vi "play-batch-raster-scan.vi"() -> ()   [LabVIEW 2017]
uses:
  raster-scan-params.ctl
  controls/PI-params.ctl
  controls/boolean_info.ctl
  controls/raster_input_meta_data.ctl
  <vilib>/userdefined/High Color/nirio_resource_hc.ctl
  controls/rasterMetaData.ctl
  <vilib>/FPGAPlugInAG/cRIO-9082/niLvFpga_Open_cRIO-9082.vi
  <vilib>/rvi/interface/common/dynamic/niFpgaDynamicAddResources.vi
  <vilib>/FPGAPlugInAG/Dynamic/niLvFpga_Reset_Dynamic.vi
  <vilib>/rvi/interface/common/niFpgaWaitOnOcc.vi
  <vilib>/Utility/error.llb/Error Cluster From Error Code.vi
  <vilib>/rvi/errors/niLvFpgaAdjustHostInterfaceError.vi
  <vilib>/FPGAPlugInAG/Dynamic/niLvFpga_Run_Dynamic.vi
  <vilib>/Utility/file.llb/Read Delimited Spreadsheet (DBL).vi
  <vilib>/FPGAPlugInAG/Dynamic/niLvFpga_Close_Dynamic.vi
  <userlib>/_matio/level5/Public/Write/Append Data Element.llb/Append Data Element (Anything).vi
  <vilib>/rvi/interface/nirviOpenFPGA/nirviOpenFPGA.xnode
  FPGA Bitfiles/afmimagingcontro_FPGATargetSPARTA_raster-scanning_DXF4O8EAjZ4.lvbitx
  <vilib>/rvi/interface/nirviMethod/nirviMethod.xnode
  <vilib>/rvi/interface/nirviReadWriteControl/nirviReadWriteControl.xnode
  <vilib>/rvi/interface/nirviCloseFPGA/nirviCloseFPGA.xnode
  <vilib>/FPGAPlugInAG/Dynamic/niLvFpga_ConfigureFifo_Dynamic.vi
  <vilib>/rvi/errors/niLvFpgaMergeErrorWithErrorCode.vi
  <vilib>/rvi/interface/Simulation/niFpgaSimulationCallBeginRW.vi
  <vilib>/FPGAPlugInAG/Dynamic/niLvFpga_ReadFifo_Dynamic.vi
  fpga_interface_lib/fpga_interface.lvlib
  NiFpgaLv.dll
  <userlib>/_matio/level5.lvlib
  <vilib>/FPGAPlugInAG/Dynamic/niLvFpga_WriteFifo_Dynamic.vi
panel:
  in  "Input-files":path[](array[path])
  out "Array 2":path[](array[path])
  out "control":dbl[](graph)
  out "error":dbl[](graph)
  out "InputMetaData":T1
  out "output-meta-data-path":path
  in  "Tab Control":enum32{"Page 1", "Debug"}(tab)
  in  "number-of-pixels":i32=256
  out "points_per_line":i32=250000
  out "total_num_points":i32
  in  "raise-constant (init)":sgl
  in  "raise-constant":sgl
  in  "trigger-0":bool
  in  "STOP":bool
  in  "xy-init":fxp<+/-,16,5>[](array[numeric])=[0.0, 0.0]
  in  "Ki-xy":dbl=0.01 format="%#_13g"
  out "ADC-zaxis":sgl
  out "DAC-zaxis":sgl
  in  "xy-bound":sgl=7.0
  out "current_output-data-path":path
  in  "note-blob":string
  in  "overwrite":bool
  in  "raster-scan-params":T2={"TsTicks"=1600, "Stop"=FALSE, "TOL"=0.3, "ramp-rate"=-5e-05, "z-u-max"=5.0, "PI-params"={"Ki"=0.01, "setpoint"=0.0}, "Num"=[1.0, 0.0, 0.0, 0.0, 0.0, 0.0, 0.0, 0.0, 0.0], "TF Order"=1, "Den"=[1.0, 0.0, 0.0, 0.0, 0.0, 0.0, 0.0, 0.0, 0.0]} {"ramp-rate" format="%#_5g"; "TOL" format="%#_13g"}
  in  "do-Dz":bool
  in  "do_xy_CL":bool
  out "boolean errors":T4
  in  "Z-settle-N":i16=10000
  out "Actual Depth":u32
  out "Elements Remaining":u32
  out "size(s)":i32
  out "y iter":i32
  out "nsamps 2":i32
  out "Empty Elements Remaining":u32
  out "(int) y*floor(x/y)":u64
  out "elements left 2":i32=1
  out "x >= y?":bool
  out "writing stopped":bool
  out "size(s) 2":i32
  out "case-selector-feedback":i16
  out "e(0) (threshhold init)":fxp<+/-,16,5>
  out "total-time":dbl
  out "x+1":i32
  out "que timed out?":bool
  out "Error signal (previous line) 2":dbl[](graph)
  out "Waveform Graph":dbl[](graph)
  out "base y_ref (ramp)":dbl[](graph)
  out "base x_ref(triangle wave)":dbl[](graph)
  out "Intensity Graph":dbl[][](graph)
  out "Error signal (previous line)":dbl[](graph)
  # "x-axis"
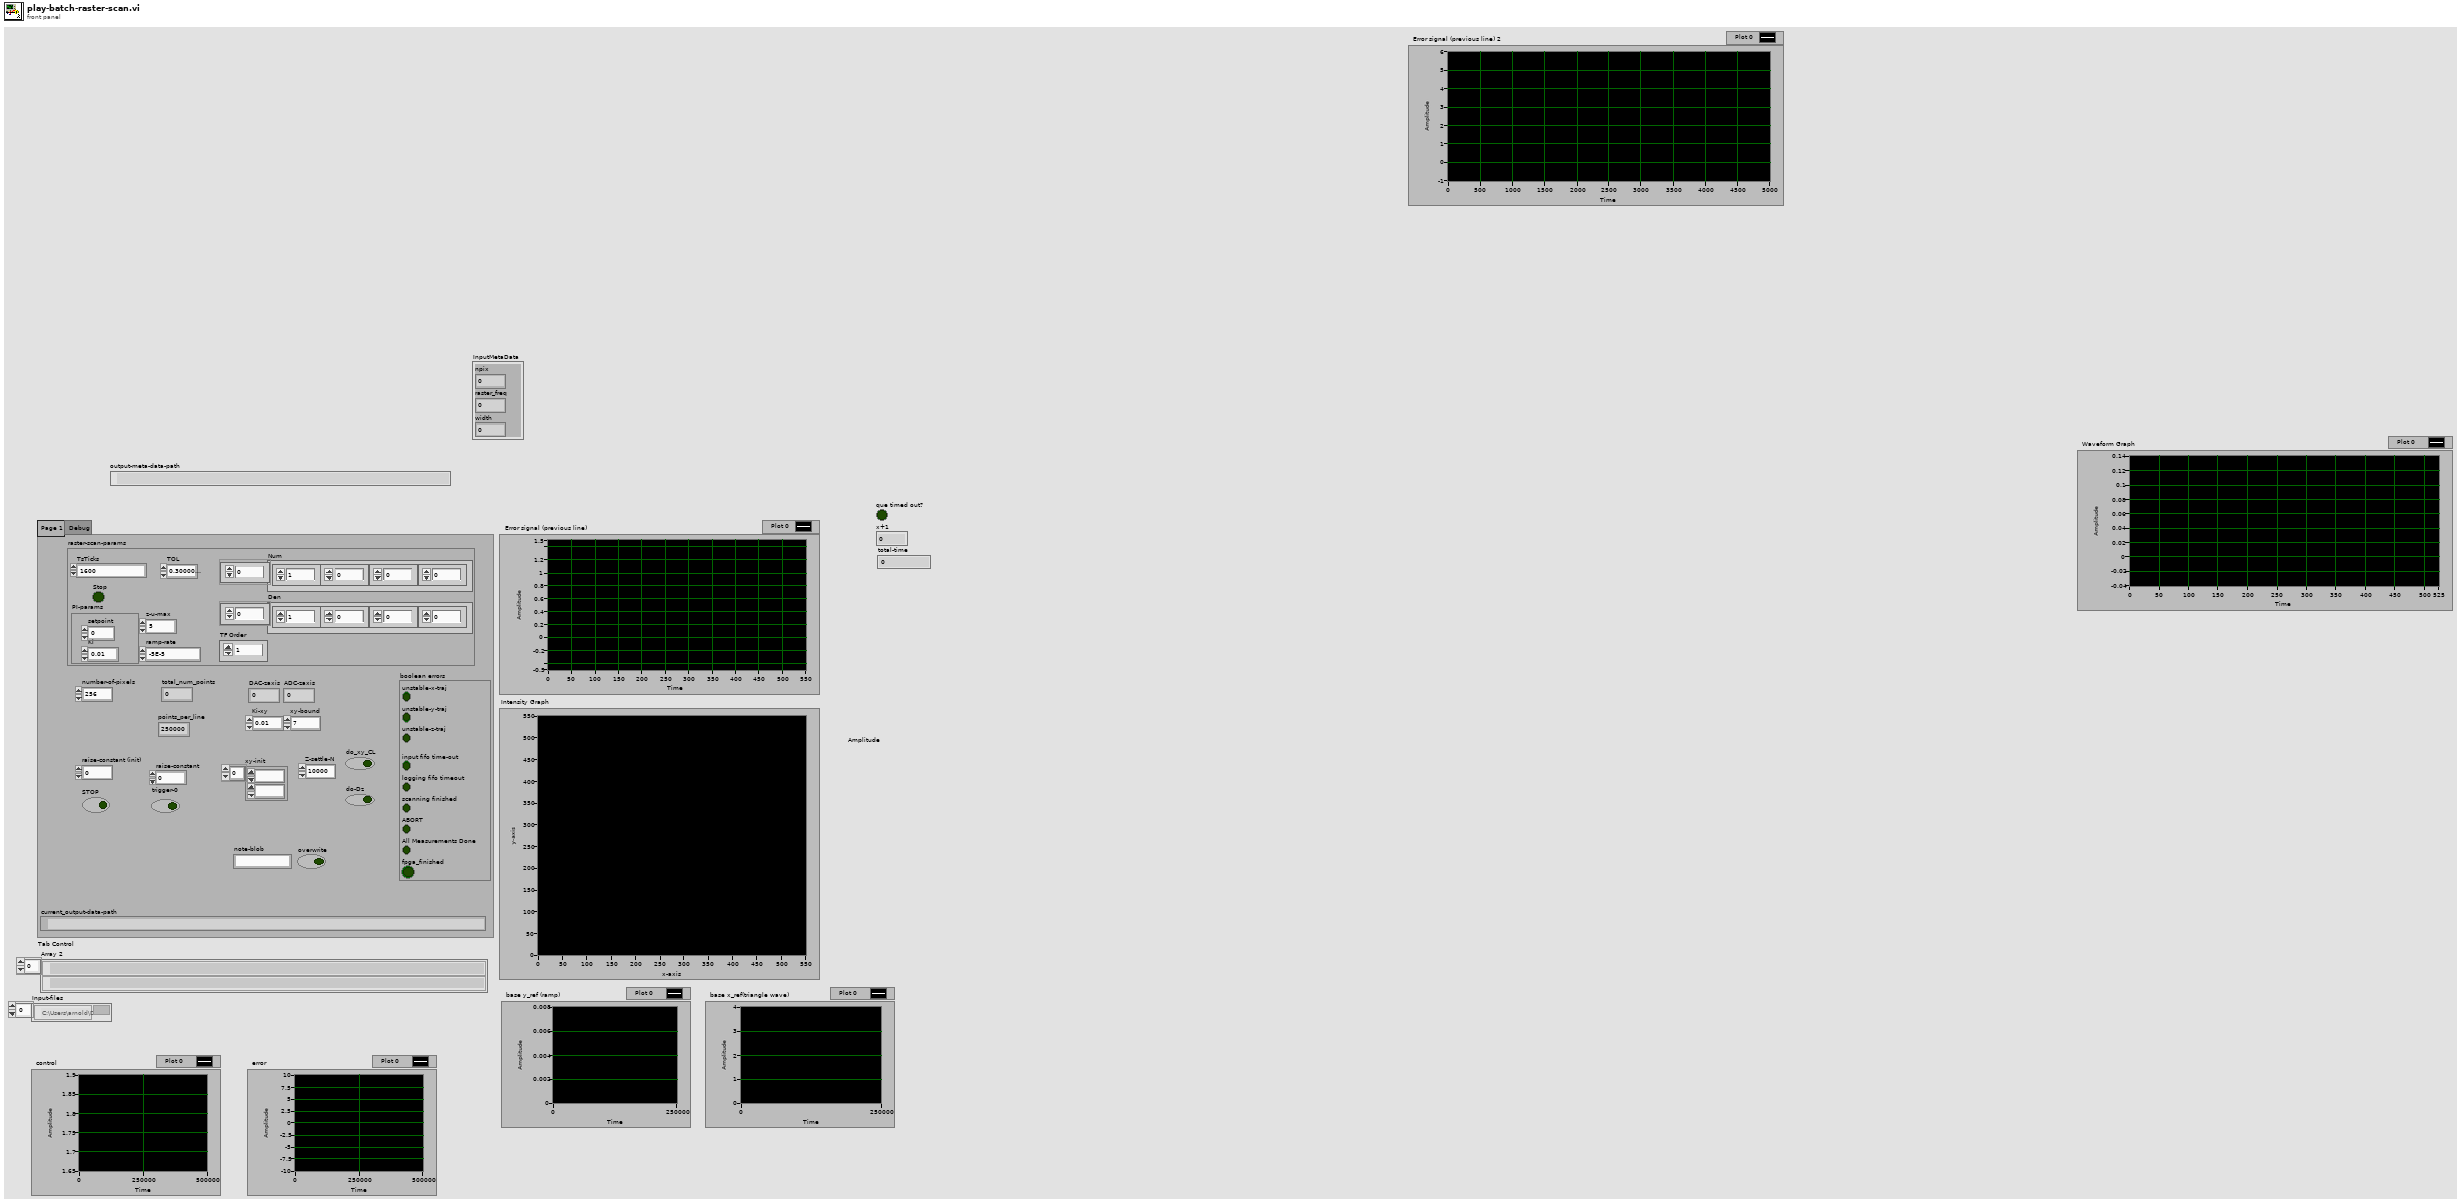
[diagram p1: front panel]
types:
  T1 = typedef "raster_input_meta_data.ctl" = cluster{"npix":dbl, "raster_freq":dbl, "width":dbl}
  T2 = typedef "raster-scan-params.ctl" = cluster{"TsTicks":u32, "Stop":bool, "TOL":sgl, "ramp-rate":sgl, "z-u-max":sgl, "PI-params":T3, "Num":sgl[], "TF Order":i32, "Den":sgl[]}
  T3 = typedef "PI-params.ctl" = cluster{"Ki":sgl, "setpoint":sgl}
  T4 = typedef "boolean_info.ctl" = cluster{"unstable-z-traj":bool, "input fifo time-out":bool, "logging fifo timeout":bool, "scanning finished":bool, "unstable-x-traj":bool, "unstable-y-traj":bool, "ABORT":bool, "All Measurements Done":bool, "fpga_finished":bool}
  T5 = typedef "nirio_resource_hc.ctl" = tag
  T6 = typedef "rasterMetaData.ctl" = cluster{"raster-scan-params":T2, "xy-bound":sgl, "DAC-zaxis":sgl, "ADC-zaxis":sgl, "Ki-xy":dbl, "total_num_points":i32, "points_per_line":i32, "number-of-lines":i32, "number-of-pixels":i32, "raster_meta_in":T1, "Ki-derate":sgl, "ze_sched_thresh":sgl}
  T7 = enum16{"open", "replace", "create", "open or create", "replace or create", "replace or create with confirmation"}
  T8 = cluster{"unstable-z-traj":bool, "input fifo time-out":bool, "logging fifo timeout":bool, "scanning finished":bool, "unstable-x-traj":bool, "unstable-y-traj":bool, "ABORT":bool, "All Measurements Done":bool, "fpga_finished":bool}
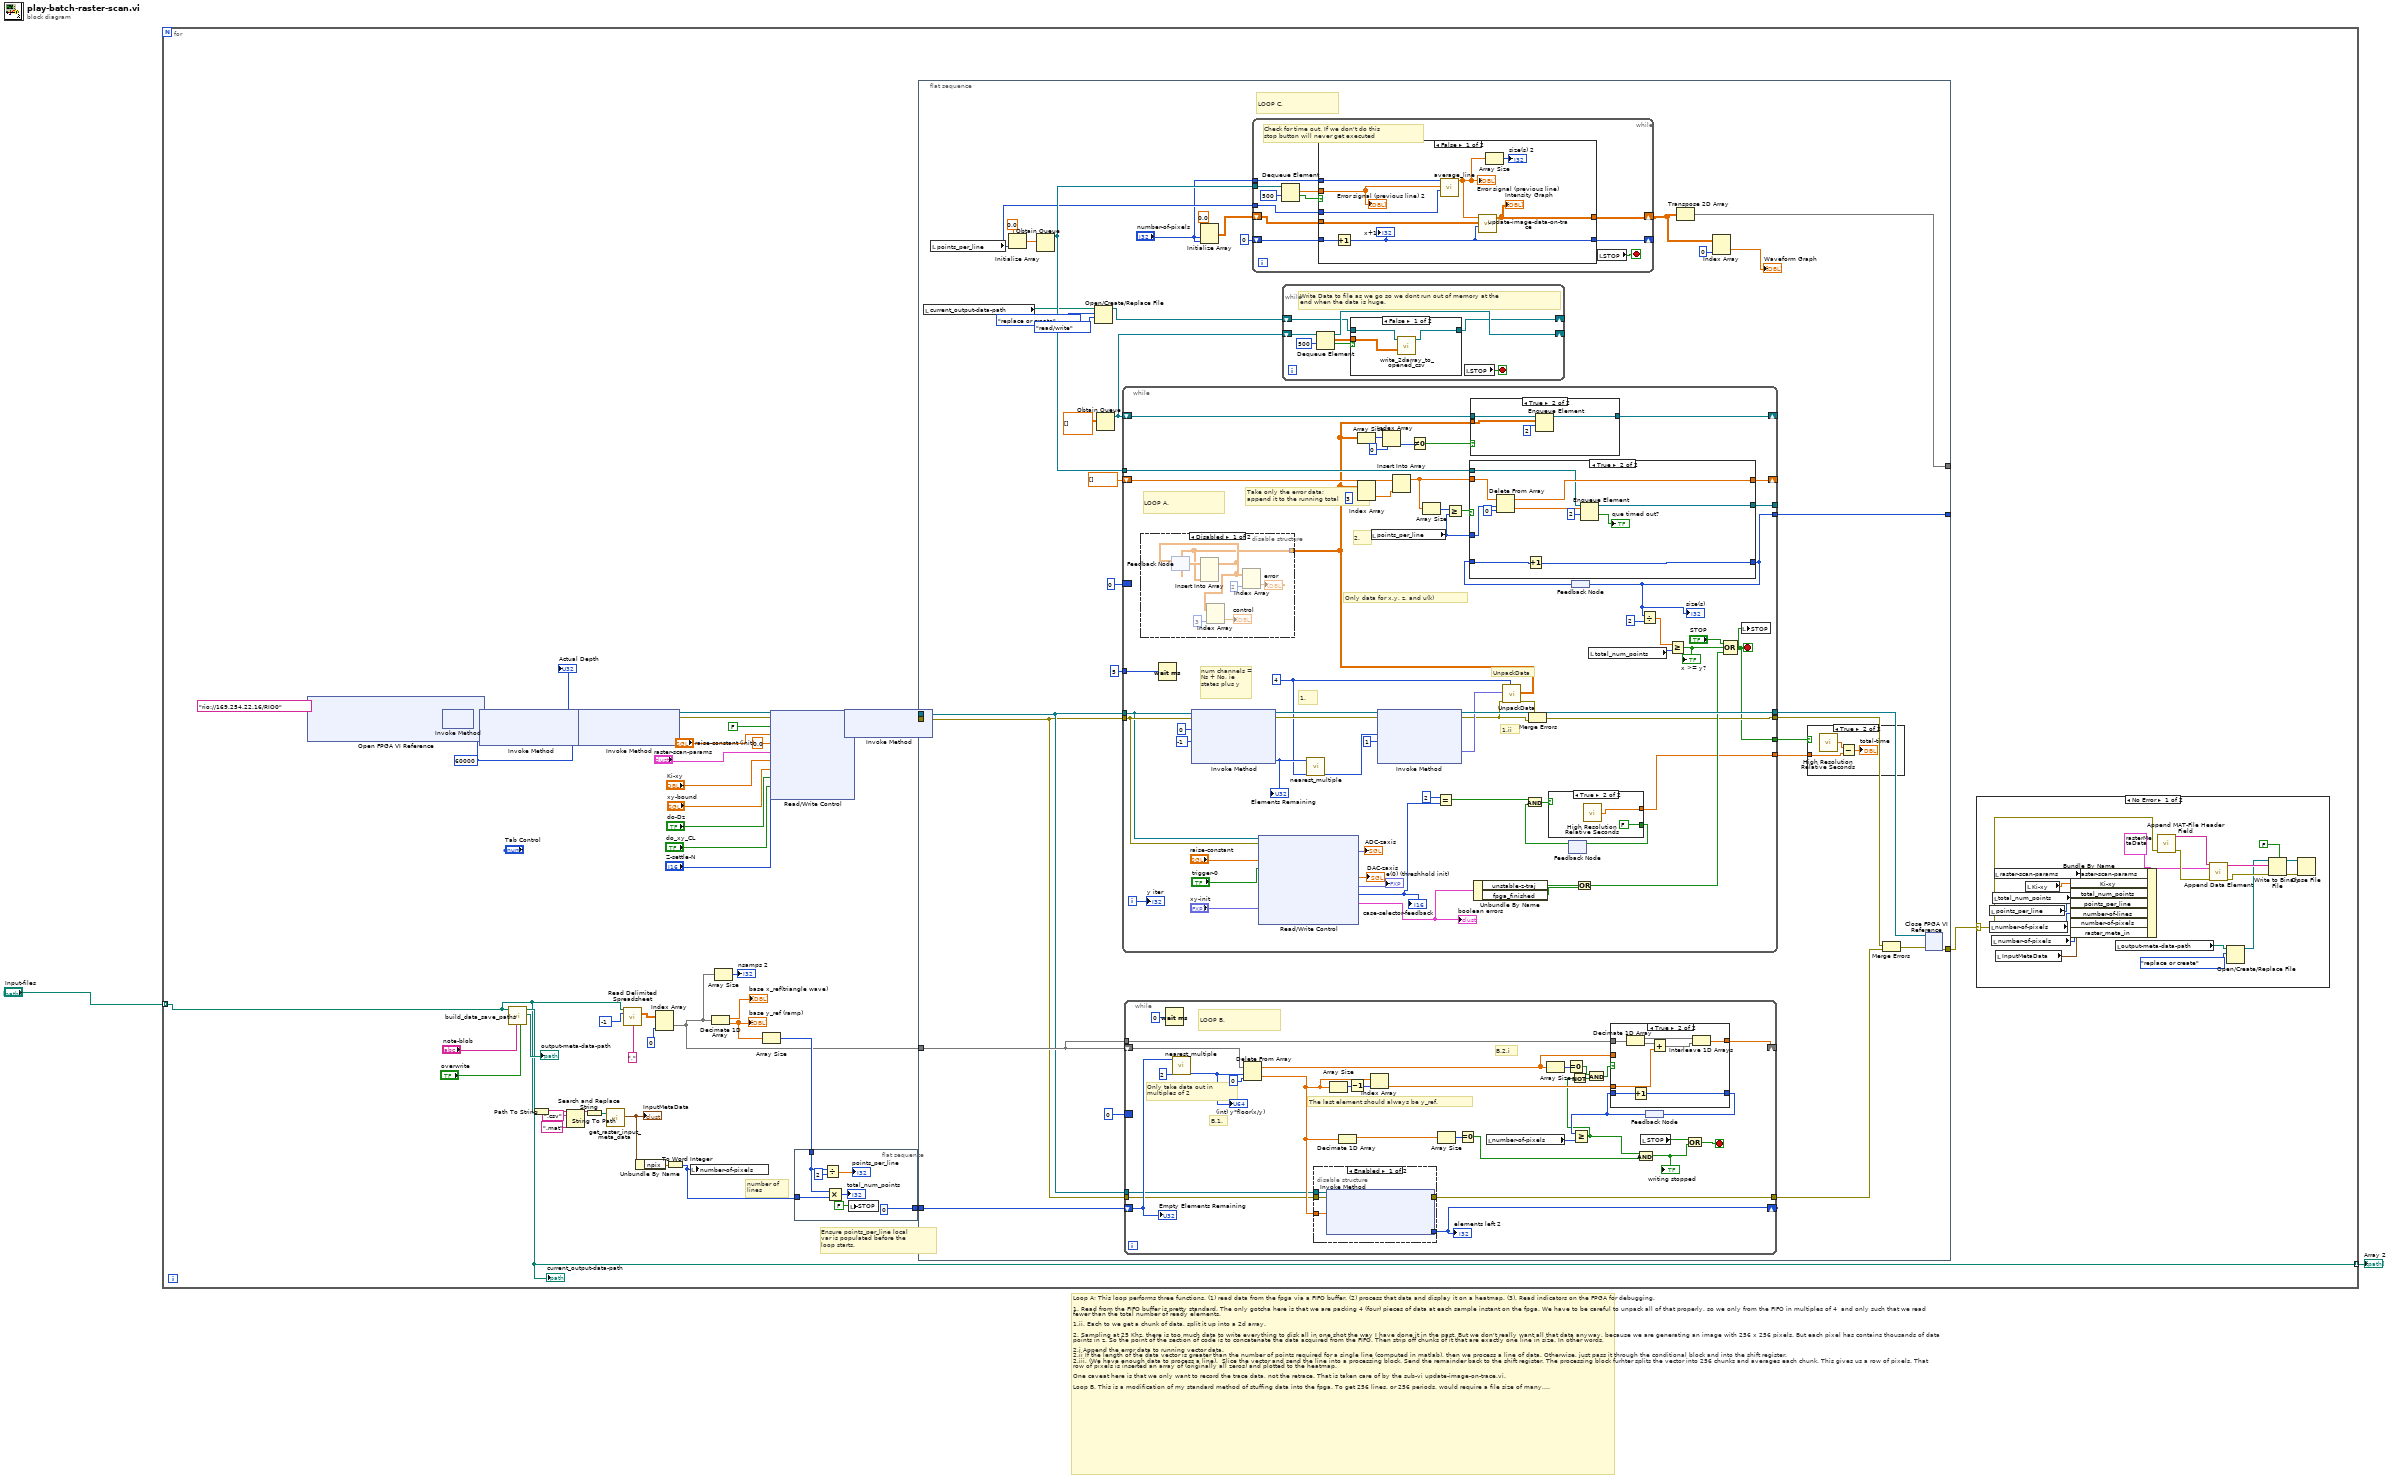
[diagram p0: block diagram]
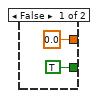
[diagram p8: hidden frame]
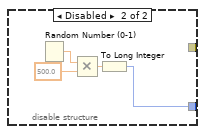
[diagram p11: hidden frame]
diagram:
  # "Loop A; This loop performs three functions. (1) read data from the fpga via a FIFO buffer. (2) process that data and display it on a heatmap. (3). Read indicators on the FPGA for debugging.\n\n1. Read from the FIFO buffer is pretty standard. The only gotcha here is that we are packing 4 (four) pieces of data at each sample instant on the fpga. We have to be careful to unpack all of that properly, so we only from the FIFO in multiples of 4  and only such that we read fewer than the total number of ready elements. \n\n1.ii. Each to we get a chunk of data, split it up into a 2d array. \n\n2. Sampling at 25 Khz, there is too much data to write everything to disk all in one shot the way I have done it in the past. But we don't really want all that data anyway, because we are generating an image with 256 x 256 pixels. But each pixel has contains thousands of data points in z. So the point of the section of code is to concatenate the data acquired from the FIFO. Then strip off chunks of it that are exactly one line in size. In other words,\n\n2.i Append the error data to running vector data.\n2.ii If the length of the data vector is greater than the number of points required for a single line (computed in matlab), then we process a line of data. Otherwise, just pass it through the conditional block and into the shift register. \n2.iii. (We have enough data to process a line).  Slice the vector and send the line into a processing block. Send the remainder back to the shift register. The processing block furhter splits the vector into 256 chunks and averages each chunk. This gives us a row of pixels. That row of pixels is inserted an array of (originally all zeros) and plotted to the heatmap.\n\nOne caveat here is that we only want to record the trace data, not the retrace. That is taken care of by the sub-vi update-image-on-trace.vi.\n\nLoop B. This is a modification of my standard method of stuffing data into the fpga. To get 256 lines, or 256 periods, would require a file size of many, many gigibtyes. SO the point here is to only use a single period of the triangle wave and corresponding ramp signal. Everytime we exauhst that data, re-cycle the same data and keep pumping it back in. The one tricky part here is that we have to be careful to shift the original ramp data up by the appropriate amount. We also have to take special care because of how the data is packed from matlab. [x(1), y(1), x(2), y(2)...].\n\nThe first iteration of the loop, we don't push any data in. All we do is get the number of empty elements.\n\nB.1 Each iteration, strip off ' empty elements ' elements from the array and send them to FIFO. \nB.2.i Is the remaining array empty?\nB.2.ii Grab the very last element. We need this"
  n1 = for {
    tunnel: [w4] -> w2 mode=indexing
    tunnel: "Input-files" -> [w3] mode=indexing
    w48 = 60000
    # "number of \nlines"
    # "Ensure points_per_line local\nvar is populated before the\nloop starts."
    n2 = xnode "Open FPGA VI Reference"("resource name"=T5 "rio://169.254.22.16/RIO0") -> ("FPGA VI Reference Out"=w47:refnum<k20>, "error out"=w46:errorcluster)  [unwired: 1 in]
    n3 = xnode "Invoke Method"("FPGA VI Reference In"=w47, "error in"=w46) -> ("FPGA VI Reference Out"=w42:refnum<k20>, "error out"=w41:errorcluster)
    n4 = xnode "Invoke Method"("FPGA VI Reference In"=w42, "error in"=w41, "Requested Depth"=w48) -> ("FPGA VI Reference Out"=w43:refnum<k20>, "error out"=w44:errorcluster, "Actual Depth"=→"Actual Depth":u32)
    n5 = call "build_data_save_paths.vi"("overwrite"="overwrite", "note-blob"="note-blob", "input-file"=w3) -> ("output-meta-data-path"=→"output-meta-data-path":path, "output-data-path"=w4:path)  [unwired: 5 in, 2 out]
    "current_output-data-path" <- w4
    n6 = Path To String(path=w3) -> (string=w12:string)
    n7 = Search and Replace String(input string=w12, search string=".csv", replace string=".mat" ("replace string (\"\")")) -> (result string=w9:string)  [unwired: 5 in, 3 out]
    n8 = xnode "Invoke Method"("FPGA VI Reference In"=w43, "error in"=w44, "Requested Depth"=w48) -> ("FPGA VI Reference Out"=w50:refnum<k20>, "error out"=w49:errorcluster)  [unwired: 1 out]
    n9 = String To Path(string=w9) -> (path=w8:path)
    n10 = call "get_raster_input_meta_data.vi"("Path"=w8) -> ("cluster"=w7:T1)  [unwired: 10 in]
    "InputMetaData" <- w7
    n11 = call-poly <vilib>:"Read Delimited Spreadsheet.vi"("file path (dialog if empty)"=w3, "number of rows (all:-1)"=-1, "delimiter (\\t)"=",") -> ("all rows"=w28:dbl[][])  [unwired: 7 in, 5 out]
    n12 = Unbundle By Name(w7) -> ("npix"=w6:dbl)
    n13 = Index Array(array=w28, index (col)=0 ("dimension size")) -> (element=w27:dbl[])  [unwired: 1 in]
    n14 = To Word Integer(number=w6) -> (16bit integer=w5:i16)
    n15 = local write "number-of-pixels"(w5) -> ()
    n16 = Decimate 1D Array(w27) -> (→"base x_ref(triangle wave)":dbl[], w34:dbl[])
    "base y_ref (ramp)" <- w34
    n17 = Array Size(array=w27) -> (size(s)=→"nsamps 2":i32)
    n18 = Array Size(array=w34) -> (size(s)=w32:i32)
    n19 = xnode "Read/Write Control"("FPGA VI Reference In"=w50, "error in"=w49, "trigger-0"=FALSE ("constant 2 lower"), "raise-constant"="raise-constant (init)", "u(0)"=sgl 0.0, "raster-scan-params"="raster-scan-params", "Ki-xy"="Ki-xy", "xy-bound"="xy-bound", "do-Dz"="do-Dz", "do_xy_CL"="do_xy_CL", "Z-settle-N"="Z-settle-N") -> ("FPGA VI Reference Out"=w24:refnum<k20>, "error out"=w23:errorcluster)
    n20 = flat-sequence {
      tunnel: [0] -> w33
      tunnel: w32 -> [w283]
      tunnel: w5 -> [w286]
      frame #0 {
        n21 = Divide(x=w283, y=2) -> (x/y=→"points_per_line":dbl)
        n22 = Multiply(x=w283, y=w286) -> (x*y=→"total_num_points":i32)
        n23 = local write "STOP"(FALSE ("STOP")) -> ()
      }
    }
    n24 = xnode "Invoke Method"("FPGA VI Reference In"=w24, "error in"=w23) -> ("FPGA VI Reference Out"=w21:refnum<k20>, "error out"=w22:errorcluster)  [unwired: 1 in]
    n25 = flat-sequence {
      tunnel: [w80] -> _
      tunnel: w21 -> [w89]
      tunnel: w22 -> [w88]
      tunnel: w33 -> [w101]
      tunnel: w27 -> [w90]
      tunnel: [w74] -> _
      tunnel: [w71] -> w16
      frame #0 {
        # "LOOP C."
        n26 = local read "current_output-data-path"() -> (w73:path)
        n27 = local read "points_per_line"() -> (w86:i32)
        n28 = Initialize Array(0.0 ("element"), w86) -> (w95:dbl[])
        n29 = Obtain Queue(element data type=w95) -> (queue out=w92:refnum<queue>)  [unwired: 4 in, 2 out]
        n30 = Open/Create/Replace File(file path (use dialog)=w73, operation (0:open)=T7."replace or create", access (0:read/write)=enum16{"read/write", "read-only", "write-only"}."read/write") -> (refnum out=w75:refnum<file>)  [unwired: 3 in, 2 out]
        n31 = Obtain Queue(element data type=dbl[][] []) -> (queue out=w78:refnum<queue>)  [unwired: 4 in, 2 out]
        n32 = while {
          tunnel: 5 -> [w200]
          tunnel: w89 -> [w191]
          tunnel: w88 -> [w192]
          tunnel: [w171] -> w83
          tunnel: [w194] -> w84
          shift-right: [w183] -> _
          shift-left: dbl[] [] -> [w181]
          border: 0 ("disabled index (col)") -> [_]
          tunnel: w92 -> [w162]
          tunnel: [w161] -> _
          tunnel: [w159] -> w82
          tunnel: [w152] -> w81
          shift-right: [w146] -> _
          shift-left: w78 -> [w145]
          tunnel: [w144] -> w74
          i -> [w190]
          stop <- w159 stop-if-true
          w168 = u32 4 ("y")
          # "2."
          # "1.ii"
          # "1."
          # "LOOP A."
          # "Take only the error data;\nappend it to the running total"
          # "num channels = Ns + No, ie states plus y"
          # "Only data for x,y, z, and u(k)"
          # "UnpackData"
          n33 = Wait (ms)(milliseconds to wait=w200) -> ()  [unwired: 1 out]
          n34 = xnode "Invoke Method"("FPGA VI Reference In"=w191, "error in"=w192, "Number of Elements"=0 ("Timeout (ms)"), "Timeout (ms)"=-1) -> ("FPGA VI Reference Out"=w196:refnum<k20>, "error out"=w197:errorcluster, "Elements Remaining"=w169:u32)  [unwired: 1 out]
          "Elements Remaining" <- w169
          n35 = xnode "Read/Write Control"("FPGA VI Reference In"=w191, "error in"=w192, "raise-constant"="raise-constant", "trigger-0"="trigger-0", "xy-init"="xy-init") -> ("ADC-zaxis"=→"ADC-zaxis":fxp<+/-,24,5>, "DAC-zaxis"=→"DAC-zaxis":sgl, "e(0) (threshhold init)"=→"e(0) (threshhold init)":fxp<+/-,16,5>, "current-case"=w158:i16, "boolean errors"=w143:T8)  [unwired: 1 in, 2 out]
          "case-selector-feedback" <- w158
          "boolean errors" <- w143
          n36 = call "nearest_multiple.vi"("numChan"=w168, "N"=w169) -> ("(int) y*floor(x/y)"=w167:u64)  [unwired: 9 in]
          n37 = local read "points_per_line"() -> (w170:i32)
          n38 = xnode "Invoke Method"("FPGA VI Reference In"=w196, "error in"=w197, "Number of Elements"=w167, "Timeout (ms)"=1) -> ("FPGA VI Reference Out"=w194:refnum<k20>, "error out"=w173:errorcluster, "Data"=w193:fxp<+/-,16,5>[])  [unwired: 1 out]
          n39 = Equal?(x=i16 2, y=w158) -> (x = y?=w156:bool)
          n40 = Unbundle By Name(w143) -> ("unstable-z-traj"=w164:bool, "fpga_finished"=w163:bool)
          n41 = call "UnpackData.vi"("NumChannels"=w168, "error In"=w173, "1D Data In"=w193) -> ("error Out"=w172:errorcluster, "2D Data Out"=w142:dbl[][])  [unwired: 7 in]
          n42 = disable-structure shown="Disabled" {
            disable-tunnel: w142 -> [w201 _]
            frame Disabled {
              n43 = feedback #1(w201) -> (w207:dbl[][])
              n44 = Insert Into Array(array=w207, new element=w201) -> (w202:dbl[][])  [unwired: 2 in]
              n45 = feedback-in #1(w202) -> ()
              n46 = Index Array(array=w202, index (col)=3 ("disabled index (col)")) -> (element=→"control":dbl[])  [unwired: 1 in]
              n47 = Index Array(array=w202, index (col)=2 ("disabled index (col)")) -> (element=→"error":dbl[])  [unwired: 1 in]
            }
            frame Enabled {
            }
          }
          n48 = Array Size(array=w142) -> (size(s)=w150:i32[])
          n49 = Index Array(array=w142, index (col)=3 ("disabled index (col)")) -> (element=w180:dbl[])  [unwired: 1 in]
          n50 = Index Array(array=w150, index=0) -> (element=w148:i32)
          n51 = Insert Into Array(array=w181, new element=w180) -> (w151:dbl[])  [unwired: 1 in]
          n52 = Not Equal To 0?(x=w148) -> (x != 0?=w147:bool)
          n53 = Array Size(array=w151) -> (size(s)=w182:i32)
          n54 = Greater Or Equal?(x=w182, y=w170) -> (x >= y?=w179:bool)
          n55 = case shown="True" w147 {
            tunnel: w145 -> [w208 w212]
            tunnel: w142 -> [_ w210]
            tunnel: [w208 w209] -> w146
            frame False {
            }
            frame True {
              n56 = Enqueue Element(queue=w212, element=w210, timeout in ms (-1)=2) -> (queue out=w209:refnum<queue>)  [unwired: 1 in, 2 out]
            }
          }
          n57 = Merge Errors(w172, w173) -> (w171:errorcluster)
          n58 = feedback #2() -> (w154:bool)  [unwired: 1 in]
          n59 = And(x=w156, y=w154) -> (x .and. y?=w157:bool)
          n60 = case shown="True" w157 {
            tunnel: [TRUE FALSE] -> w155
            tunnel: [0.0 ("relative seconds") w215] -> w152
            frame False {
            }
            frame True {
              n61 = call <vilib>:"High Resolution Relative Seconds.vi"() -> ("relative seconds"=w215:dbl)
            }
          }
          n62 = feedback-in #2(w155) -> ()
          n63 = feedback #3() -> (w178:i32)
          n64 = case shown="True" w179 {
            tunnel: [w219 w228] -> w183
            tunnel: w151 -> [w219 w230]
            tunnel: w178 -> [w218 w227]
            tunnel: [w218 w226] -> w144
            tunnel: w170 -> [_ w225]
            tunnel: w162 -> [w217 w223]
            tunnel: [w217 w222] -> w161
            frame False {
            }
            frame True {
              n65 = Delete From Array(array=w230, length=w225, index=0) -> (deleted portion=w224:dbl[], array with subset deleted=w228:dbl[])
              n66 = Increment(x=w227) -> (x+1=w226:i32)
              n67 = Enqueue Element(queue=w223, element=w224, timeout in ms (-1)=2) -> (queue out=w222:refnum<queue>, timed out?=→"que timed out?":bool)  [unwired: 1 in, 1 out]
            }
          }
          "size(s)" <- w144
          n68 = feedback-in #3(w144) -> ()
          n69 = Or(x=w164, y=w163) -> (x .or. y?=w174:bool)
          n70 = local read "total_num_points"() -> (w177:i32)
          n71 = Divide(x=w144, y=2) -> (x/y=w166:dbl)
          n72 = Greater Or Equal?(x=w166, y=w177) -> (x >= y?=w175:bool)
          "x >= y?" <- w175
          n73 = Compound Arithmetic op=OR("STOP", w175, w174) -> (w159:bool)
          n74 = local write "STOP"(w159) -> ()
          "y iter" <- w190
        }
        n75 = while {
          shift-right: [w260] -> _
          shift-left: w101 -> [w255]
          shift-right: [w248] -> _
          shift-left: w90 -> [w261]
          tunnel: w90 -> [w246]
          tunnel: [w252] -> w102
          tunnel: w89 -> [w244]
          tunnel: w88 -> [w243]
          border: 0 ("Timeout (ms)") -> [_]
          stop <- w256 stop-if-true
          # "B.2.i"
          # "B.1."
          # "LOOP B."
          # "Only take data out in \nmultiples of 2"
          # "The last element should always be y_ref."
          n76 = Wait (ms)(milliseconds to wait=0) -> ()  [unwired: 1 out]
          n77 = call "nearest_multiple.vi"("numChan"=u32 2 ("Empty Elements Remaining"), "N"=w255) -> ("(int) y*floor(x/y)"=w254:u64)  [unwired: 9 in]
          "(int) y*floor(x/y)" <- w254
          n78 = Delete From Array(array=w261, length=w254, index=0) -> (deleted portion=w249:dbl[], array with subset deleted=w247:dbl[])
          n79 = disable-structure shown="Enabled" {
            disable-tunnel: [w276 w277] -> w260
            disable-tunnel: w249 -> [w275 _]
            disable-tunnel: [w274 _] -> w252
            disable-tunnel: w244 -> [w273 _]
            disable-tunnel: w243 -> [w272 _]
            frame Enabled {
              n80 = xnode "Invoke Method"("FPGA VI Reference In"=w273, "error in"=w272, "Data"=w275) -> ("error out"=w274:errorcluster, "Empty Elements Remaining"=w276:u32)  [unwired: 1 in, 1 out]
            }
            frame Disabled {
              n81 = Random Number (0-1)() -> (number: 0 to 1=w280:dbl)
              n82 = Multiply(x=w280, y=500.0) -> (x*y=w278:dbl)
              n83 = To Long Integer(number=w278) -> (32bit integer=w277:i32)
            }
          }
          "elements left 2" <- w260
          n84 = Array Size(array=w249) -> (size(s)=w250:i32)
          n85 = Decimate 1D Array(w249) -> (w235:dbl[])  [unwired: 1 out]
          n86 = Decrement(x=w250) -> (x-1=w251:i32)
          n87 = Index Array(array=w249, index=w251) -> (element=w245:dbl)
          n88 = Array Size(array=w235) -> (size(s)=w237:i32)
          n89 = Equal To 0?(x=w237) -> (x = 0?=w236:bool)
          n90 = local read "number-of-pixels"() -> (w241:i32)
          n91 = Array Size(array=w247) -> (size(s)=w258:i32)
          n92 = Equal To 0?(x=w258) -> (x = 0?=w234:bool)
          n93 = local read "STOP"() -> (w257:bool)
          n94 = feedback #4() -> (w239:i32)
          n95 = Greater Or Equal?(x=w239, y=w241) -> (x >= y?=w232:bool)
          n96 = Not(x=w232) -> (.not. x?=w233:bool)
          n97 = And(x=w234, y=w233) -> (x .and. y?=w231:bool)
          n98 = case shown="True" w231 {
            tunnel: [w263 w266] -> w248
            tunnel: w247 -> [w263 _]
            tunnel: w246 -> [_ w271]
            tunnel: w245 -> [_ w269]
            tunnel: [w262 w265] -> w240
            tunnel: w239 -> [w262 w264]
            frame False {
            }
            frame True {
              n99 = Decimate 1D Array(w271) -> (w268:dbl[], w270:dbl[])
              n100 = Increment(x=w264) -> (x+1=w265:i32)
              n101 = Add(x=w270, y=w269) -> (x+y=w267:dbl[])
              n102 = Interleave 1D Arrays(w268, w267) -> (w266:dbl[])
            }
          }
          n103 = And(x=w232, y=w236) -> (x .and. y?=w238:bool)
          "writing stopped" <- w238
          n104 = feedback-in #4(w240) -> ()
          n105 = Or(x=w257, y=w238) -> (x .or. y?=w256:bool)
          "Empty Elements Remaining" <- w255
        }
        n106 = Initialize Array(0.0 ("element"), "number-of-pixels", "number-of-pixels") -> (w94:dbl[][])
        n107 = while {
          shift-right: [w130] -> w91
          shift-left: w94 -> [w129]
          shift-right: [w127] -> _
          shift-left: 0 ("disabled index (col)") -> [w128]
          tunnel: w86 -> [w126]
          tunnel: w92 -> [w125]
          tunnel: "number-of-pixels" -> [w120]
          stop <- w123 stop-if-true
          # "Check for time out. If we don't do this\nstop button will never get executed"
          n108 = Dequeue Element(queue=w125, timeout in ms (-1)=500) -> (element=w124:dbl[], timed out?=w121:bool)  [unwired: 1 in, 2 out]
          n109 = case shown="False" w121 {
            tunnel: [w139 w140] -> w130
            tunnel: w129 -> [w138 w140]
            tunnel: w128 -> [w137 w141]
            tunnel: [w136 w141] -> w127
            tunnel: w126 -> [w135 _]
            tunnel: w124 -> [w134 _]
            tunnel: w120 -> [w131 _]
            frame False {
              n110 = Increment(x=w137) -> (x+1=w136:i32)
              "x+1" <- w136
              n111 = call "average_line.vi"("data-pts-per-line"=w135, "raw-data-row"=w134, "number-of-pixels"=w131) -> ("avg-data-row"=w133:dbl[])  [unwired: 8 in]
              "Error signal (previous line)" <- w133
              n112 = call "update-image-data-on-trace.vi"("iterator"=w136, "master-image-data-n"=w138, "avg-data-row"=w133) -> ("master-image-data-out"=w139:dbl[][])  [unwired: 8 in]
              "Intensity Graph" <- w139
              n113 = Array Size(array=w133) -> (size(s)=→"size(s) 2":i32)
              "Error signal (previous line) 2" <- w134
            }
            frame True {
            }
          }
          n114 = local read "STOP"() -> (w123:bool)
        }
        n115 = while {
          shift-right: [w107] -> _
          shift-left: w78 -> [w108]
          shift-right: [w105] -> _
          shift-left: w75 -> [w106]
          stop <- w110 stop-if-true
          # "Write Data to file as we go so we dont run out of memory at the \nend when the data is huge."
          n116 = Dequeue Element(queue=w108, timeout in ms (-1)=500) -> (queue out=w107:refnum<queue>, element=w109:dbl[][], timed out?=w111:bool)  [unwired: 1 in, 1 out]
          n117 = case shown="False" w111 {
            tunnel: w109 -> [w113 _]
            tunnel: w106 -> [w115 w116]
            tunnel: [w114 w116] -> w105
            frame False {
              n118 = call "write_2darray_to_opened_csv.vi"("Data_in"=w113, "file_ref_in"=w115) -> ("file_ref_out"=w114:refnum<file>)  [unwired: 9 in]
            }
            frame True {
            }
          }
          n119 = local read "STOP"() -> (w110:bool)
        }
        n120 = Transpose 2D Array(2D array=w91) -> (transposed array=w80:dbl[][])
        n121 = Index Array(array=w91, index (col)=0 ("disabled index (col)")) -> (element=→"Waveform Graph":dbl[])  [unwired: 1 in]
        n122 = case shown="True" w82 {
          tunnel: w81 -> [_ w119]
          frame False {
          }
          frame True {
            n123 = call <vilib>:"High Resolution Relative Seconds.vi"() -> ("relative seconds"=w118:dbl)
            n124 = Subtract(x=w118, y=w119) -> (x-y=→"total-time":dbl)
          }
        }
        n125 = Merge Errors(w83, w102) -> (w72:errorcluster)
        n126 = xnode "Close FPGA VI Reference"("FPGA VI Reference In"=w84, "error in"=w72) -> ("error out"=w71:errorcluster)
      }
    }
    n127 = case shown="No Error" w16 {
      selector: w16 -> [w59 _]
      frame No Error {
        n128 = local read "number-of-pixels"() -> (w53:i32)
        n129 = local read "points_per_line"() -> (w54:i32)
        n130 = local read "number-of-pixels"() -> (w52:i32)
        n131 = local read "total_num_points"() -> (w55:i32)
        n132 = local read "raster-scan-params"() -> (w57:T2)
        n133 = local read "InputMetaData"() -> (w51:T1)
        n134 = local read "Ki-xy"() -> (w56:dbl)
        n135 = Bundle By Name(cluster=T6 {"raster-scan-params"={"TsTicks"=1600, "Stop"=TRUE, "TOL"=0.3, "ramp-rate"=-5e-05, "z-u-max"=5.0, "PI-params"={"Ki"=0.01, "setpoint"=0.0}, "Num"=[1.0, 0.0, 0.0, 0.0, 0.0, 0.0, 0.0, 0.0, 0.0], "TF Order"=3, "Den"=[1.0, 0.0, 0.0, 0.0, 0.0, 0.0, 0.0, 0.0, 0.0]}, "xy-bound"=7.0, "DAC-zaxis"=0.0, "ADC-zaxis"=0.0, "Ki-xy"=0.01, "total_num_points"=0, "points_per_line"=250000, "number-of-lines"=256, "number-of-pixels"=256, "raster_meta_in"={"npix"=0.0, "raster_freq"=0.0, "width"=0.0}, "Ki-derate"=0.01, "ze_sched_thresh"=0.0} ("Cluster"), "raster-scan-params"=w57, "Ki-xy"=w56, "total_num_points"=w55, "points_per_line"=w54, "number-of-lines"=w53, "number-of-pixels"=w52, "raster_meta_in"=w51) -> (w58:T6)
        n136 = local read "output-meta-data-path"() -> (w61:path)
        n137 = call <userlib>:"Append MAT-File Header Field.vi"("error"=w59) -> ("result string"=w70:string, "error out"=w64:errorcluster)  [unwired: 13 in]
        n138 = call-poly <userlib>:"Append Data Element.vi"("initial string"=w70, "data"=w58, "error in (no error)"=w64) -> ("result string"=w68:string, "error out"=w69:errorcluster)  [unwired: 11 in]
        n139 = Open/Create/Replace File(file path (use dialog)=w61, operation (0:open)=T7."replace or create") -> (refnum out=w63:refnum<file>)  [unwired: 4 in, 2 out]
        n140 = Write to Binary File(file (use dialog)=w63, data=w68, error in=w69, 5:FALSE ("prepend array or string size? (T)")) -> (refnum out=w65:refnum<file>, error out=w66:errorcluster)  [unwired: 2 in, 1 out]
        n141 = Close File(refnum=w65, error in=w66) -> ()  [unwired: 2 out]
      }
      frame Error {
      }
    }
  }
  "Array 2" <- w2
